vi "Simple Solenoid - Test.vi"() -> ()   [LabVIEW 2019]
uses:
  <vilib>/Rock Robotics/WPI/Solenoid/WPI_SolenoidValue.ctl
  <vilib>/Rock Robotics/WPI/Solenoid/WPI_SolenoidChannel.ctl
  <vilib>/Rock Robotics/WPI/Solenoid/WPI_SolenoidOpenDouble.vi
  <vilib>/Rock Robotics/WPI/Solenoid/WPI_SolenoidSetEnum.vi
  <vilib>/Rock Robotics/WPI/Joystick/WPI_JoystickDeviceEnum.ctl
panel:
  in  "Joystick Port":T1
  in  "stop":bool
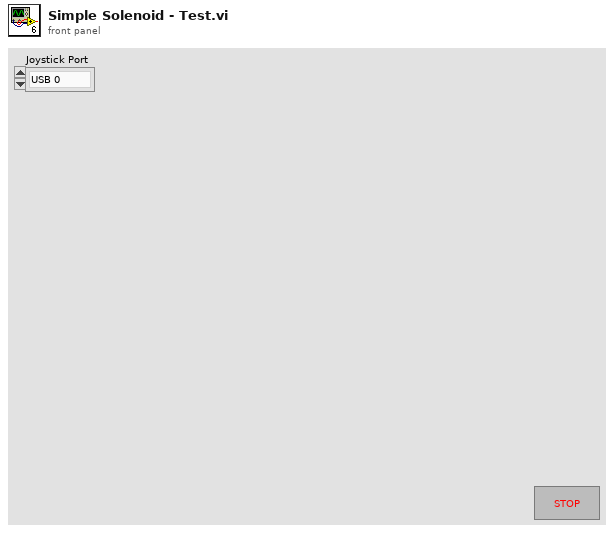
[diagram p1: front panel]
types:
  T1 = typedef "WPI_JoystickDeviceEnum.ctl" = enum16{"USB 0", "USB 1", "USB 2", "USB 3", "USB 4", "USB 5"}
  T2 = typedef "WPI_SolenoidChannel.ctl" = enum8{"Solenoid 0", "Solenoid 1", "Solenoid 2", "Solenoid 3", "Solenoid 4", "Solenoid 5", "Solenoid 6", "Solenoid 7", "Invalid"}
  T3 = typedef "WPI_JoystickDevRef.ctl" = cluster{"Device":T1}
  T4 = typedef "WPI_SolenoidDevRef.ctl" = cluster{"DevStatus":errorcluster, "Pneumatics Control Module":u8, "Forward Solenoid Channel":T2, "Reverse Solenoid Channel":T2}
  T5 = typedef "WPI_SolenoidValue.ctl" = enum16{"Off", "On", "Forward", "Reverse"}
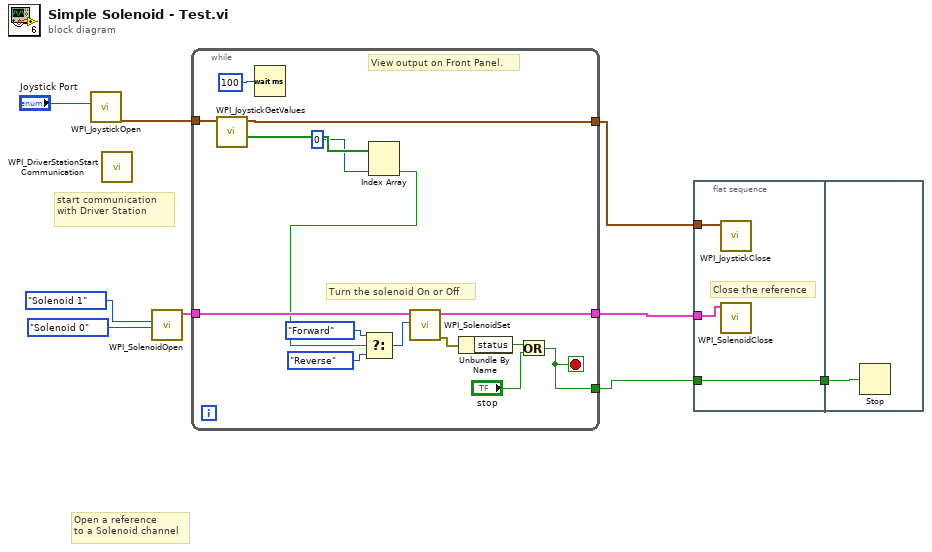
[diagram p0: block diagram]
diagram:
  # "start communication with Driver Station"
  # "Open a reference \nto a Solenoid channel"
  n1 = call <vilib>:"WPI_JoystickOpen.vi"("JoystickDevice"="Joystick Port") -> ("JoystickDevRef"=w4:T3)  [unwired: 10 out]
  n2 = call <vilib>:"WPI_DriverStationStart Communication.vi"() -> ()  [unwired: 2 in, 10 out]
  n3 = call-poly <vilib>:"WPI_SolenoidOpen.vi"("Reverse Solenoid Channel"=WPI_SolenoidChannel."Solenoid 0", "Forward Solenoid Channel"=WPI_SolenoidChannel."Solenoid 1") -> ("SolenoidDevRef"=w9:T4)  [unwired: 2 in, 7 out]
  n4 = while {
    tunnel: w9 -> [w23]
    tunnel: [w22] -> w1
    tunnel: [w18] -> w8
    tunnel: w4 -> [w14]
    tunnel: [w13] -> w2
    stop <- w18 stop-if-true
    # "View output on Front Panel."
    # "Turn the solenoid On or Off"
    n5 = call <vilib>:"WPI_JoystickGetValues.vi"("JoystickDevRef"=w14) -> ("Buttons"=w12:bool[], "JoystickDevRef"=w13:T3)  [unwired: 6 in, 3 out]
    n6 = Wait (ms)(milliseconds to wait=u32 100) -> ()  [unwired: 1 out]
    n7 = Index Array(array=w12, index #2=0 ("index")) -> (element #2=w10:bool)  [unwired: 1 in, 1 out]
    n8 = Select(t=WPI_SolenoidValue."Forward" ("Value"), s=w10, f=WPI_SolenoidValue."Reverse" ("Value")) -> (s? t:f=w15:T5)
    n9 = call-poly <vilib>:"WPI_SolenoidSet.vi"("Value"=w15, "SolenoidDevRef"=w23) -> ("error out"=w21:errorcluster, "SolenoidDevRef"=w22:T4)  [unwired: 1 in, 7 out]
    n10 = Unbundle By Name(w21) -> ("status"=w20:bool)
    n11 = Or(x=w20, y="stop") -> (x .or. y?=w18:bool)
  }
  n12 = flat-sequence {
    tunnel: w8 -> [w27]
    tunnel: [w27] -> w3
    tunnel: w2 -> [w26]
    tunnel: w1 -> [w25]
    tunnel: w3 -> [w28]
    frame #0 {
      # "Close the reference"
      n13 = call <vilib>:"WPI_JoystickClose.vi"("JoystickDevRef"=w26) -> ()  [unwired: 11 out]
      n14 = call <vilib>:"WPI_SolenoidClose.vi"("SolenoidDevRef"=w25) -> ()  [unwired: 1 in, 10 out]
    }
    frame #1 {
      n15 = Stop(stop? (T)=w28) -> ()
    }
  }
